vi "List All PPL Classes.vi"(7 "Force reload?(F)":bool) -> (2 "PPL Class File Names":string[](array[string]), 3 "PPL Class Paths":path[](array[path]))   [LabVIEW 2020, in "Utility.lvlib"]
doc: "Find and return (and store on a feedback node) all classes in the PPL folder."
uses:
  Utility.lvlib
  <vilib>/Utility/LVLibp/NI_PackedLibraryUtility.lvlib
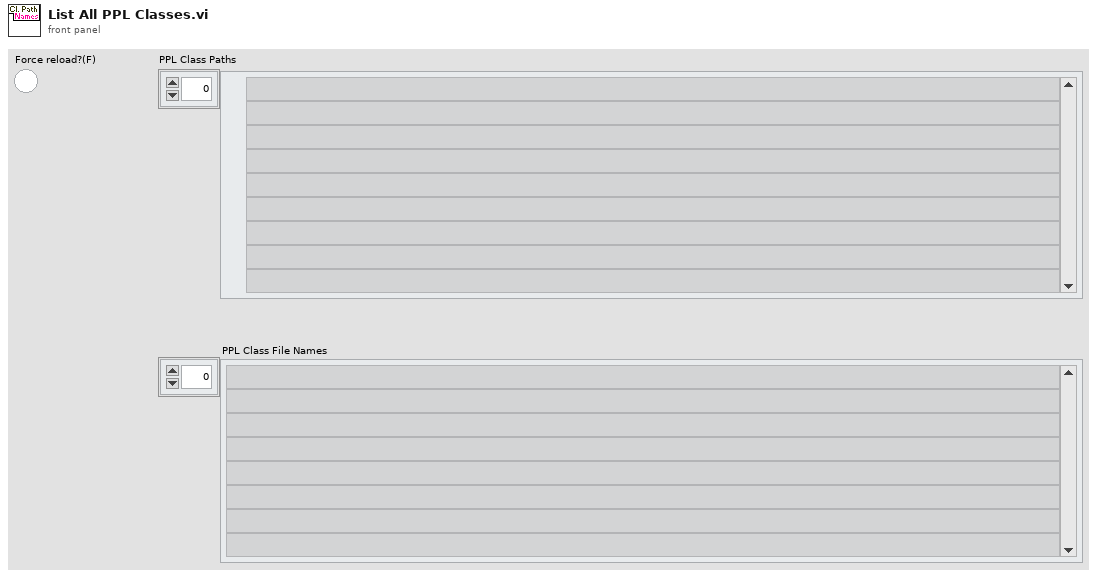
[diagram p1: front panel]
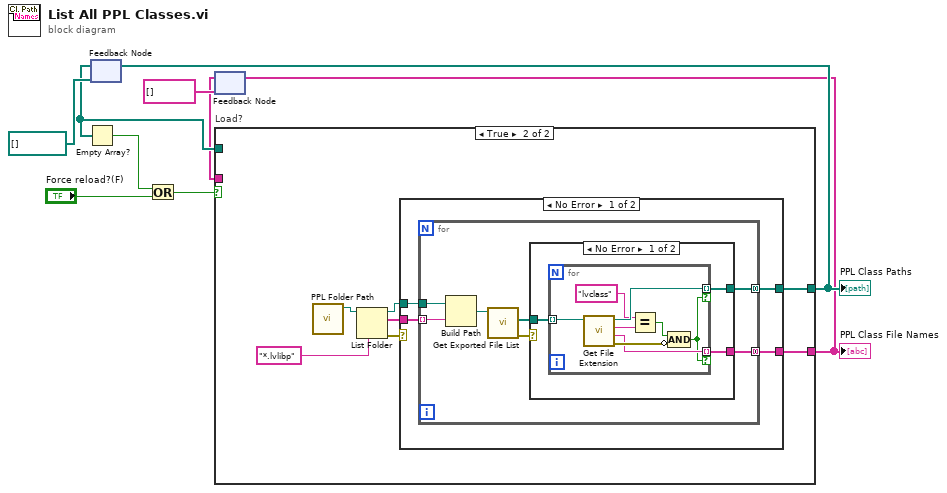
[diagram p0: block diagram]
diagram:
  n1 = feedback #1(path[] [] ("PPL Class Paths")) -> (w5:path[])
  n2 = Empty Array?(array=w5) -> (empty?=w8:bool)
  n3 = Or(x=w8, y="Force reload?(F)") -> (x .or. y?=w6:bool)
  n4 = feedback #2(string[] []) -> (w1:string[])
  n5 = case "Load?" shown="True" w6 {
    tunnel: [w11 w14] -> w4
    tunnel: w5 -> [w11 _]
    tunnel: [w10 w12] -> w2
    tunnel: w1 -> [w10 _]
    frame False {
    }
    frame True {
      n6 = call "PPL Folder Path.vi"() -> ("PPL Folder Path"=w13:path)  [unwired: 11 in]
      n7 = List Folder(path=w13, pattern="*.lvlibp") -> (path out=w15:path, filenames=w16:string[], error out=w17:errorcluster)  [unwired: 2 in, 1 out]
      n8 = case shown="No Error" w17 {
        tunnel: w16 -> [w21 _]
        tunnel: w15 -> [w22 _]
        tunnel: [w20 _] -> w14
        tunnel: [w19 _] -> w12
        frame No Error {
          n9 = for {
            tunnel: w22 -> [w29]
            tunnel: w21 -> [w28] mode=indexing
            tunnel: [w25] -> w20 mode=concatenating
            tunnel: [w23] -> w19 mode=concatenating
            n10 = Build Path(base path=w29, name or relative path=w28) -> (appended path=w27:path)
            n11 = call <vilib>:"Get Exported File List.vi"("packed library path"=w27) -> ("error out"=w24:errorcluster, "paths"=w26:path[])  [unwired: 8 in, 1 out]
            n12 = case shown="No Error" w24 {
              tunnel: w26 -> [w32 _]
              tunnel: [w31 _] -> w25
              tunnel: [w30 _] -> w23
              frame No Error {
                n13 = for {
                  tunnel: w32 -> [w40] mode=indexing
                  tunnel: [w39] -> w31 mode=indexing if=w33
                  tunnel: [w34] -> w30 mode=indexing if=w33
                  n14 = call <vilib>:"Get File Extension.vi"("file"=w40) -> ("error out"=w35:errorcluster, "filename without extension"=w34:string, "lowercase file extension"=w38:string, "dup file"=w39:path)  [unwired: 6 in, 1 out]
                  n15 = Equal?(x="lvclass" ("y"), y=w38) -> (x = y?=w36:bool)
                  n16 = Compound Arithmetic op=AND(w36, invert w35) -> (w33:bool)
                }
              }
              frame Error {
              }
            }
          }
        }
        frame Error {
        }
      }
    }
  }
  "PPL Class Paths" <- w4
  "PPL Class File Names" <- w2
  n17 = feedback-in #1(w4) -> ()
  n18 = feedback-in #2(w2) -> ()
